vi "Settings Dialog.vi"(8 "error in (no error)":errorcluster, 11 "Settings in":T3={"Acquisition"={"State"=enum."Idle S3DK", "Settings"="", "Online"=FALSE, "S3DK"={"Signals"={"Phasor"=[], "Analog"=[], "Digital"=[]}}, "CSV"={"Index"=0, "Parcel Length"=0, "EOF?"=FALSE, "Config"={"Mode"=enum."Full timestamp", "delimiter (\\t)"="\t", "Path"=path "", "Rectangular?"=FALSE}}}, "Logging"={"Logging State"=enum."Idle", "Settings"="", "Buffer"={"Index"=0, "Size"=15000, "Samples"=0, "Ordered ?"=FALSE}}, "Processing"={"Settings"="", "Parameters"={"Index"=0, "Size"=0, "Samples"=0, "Ordered ?"=FALSE}, "Refresh Rate"=0}}) -> (0 "error out":errorcluster, 1 "Changed?":bool, 2 "UI Refresh Needed?":bool, 3 "Settings out":T3={"Acquisition"={"State"=enum."Idle S3DK", "Settings"="", "Online"=FALSE, "S3DK"={"Signals"={"Phasor"=[], "Analog"=[], "Digital"=[]}}, "CSV"={"Index"=0, "Parcel Length"=0, "EOF?"=FALSE, "Config"={"Mode"=enum."Full timestamp", "delimiter (\\t)"="\t", "Path"=path "", "Rectangular?"=FALSE}}}, "Logging"={"Logging State"=enum."Idle", "Settings"="", "Buffer"={"Index"=0, "Size"=15000, "Samples"=0, "Ordered ?"=FALSE}}, "Processing"={"Settings"="", "Parameters"={"Index"=0, "Size"=0, "Samples"=0, "Ordered ?"=FALSE}, "Refresh Rate"=0}})   [LabVIEW 2017, in "Settings.lvlib"]
doc: "Dialog for selecting user specified settings."
uses:
  Settings.lvlib
  Settings.ctl
  acquisition/Acquisition Settings.ctl
  acquisition/Acquisition State.ctl
  libs/CSV Reader/Mode CSV reader.ctl
  logging/Logging Configuration.ctl
  logging/Logging State.ctl
  libs/PMU Buffer/Buffer Settings.ctl
  processing/Processing Settings.ctl
  acquisition/Acquisition.lvlib
  logging/Logging.lvlib
  processing/Processing.lvlib
  libs/PMU Buffer/PMU data buffer.lvlib
panel:
  in  "Restore Default":bool
  in  "CSV":T2={"Mode"=enum."Full timestamp", "delimiter (\\t)"=";", "Path"=path "", "Rectangular?"=FALSE}
  in  "Online?":bool
  in  "Parcel Length":i32=20
  in  "Refresh Rate":u32(ring)=1000 caption="Hz" items=["1"=1000, "5"=200, "10"=100, "25"=40, "50"=20]
  in  "Buffer Size":i32=3000
  in  "Cancel Button":bool
  in  "OK Button":bool
  # "Non visible portion of dialog (needed for connector pane)."
  # "Buffer Paremeters"
  # "Buffer Paremeters"
  # "Buffer Paremeters"
  # "Buffer Paremeters"
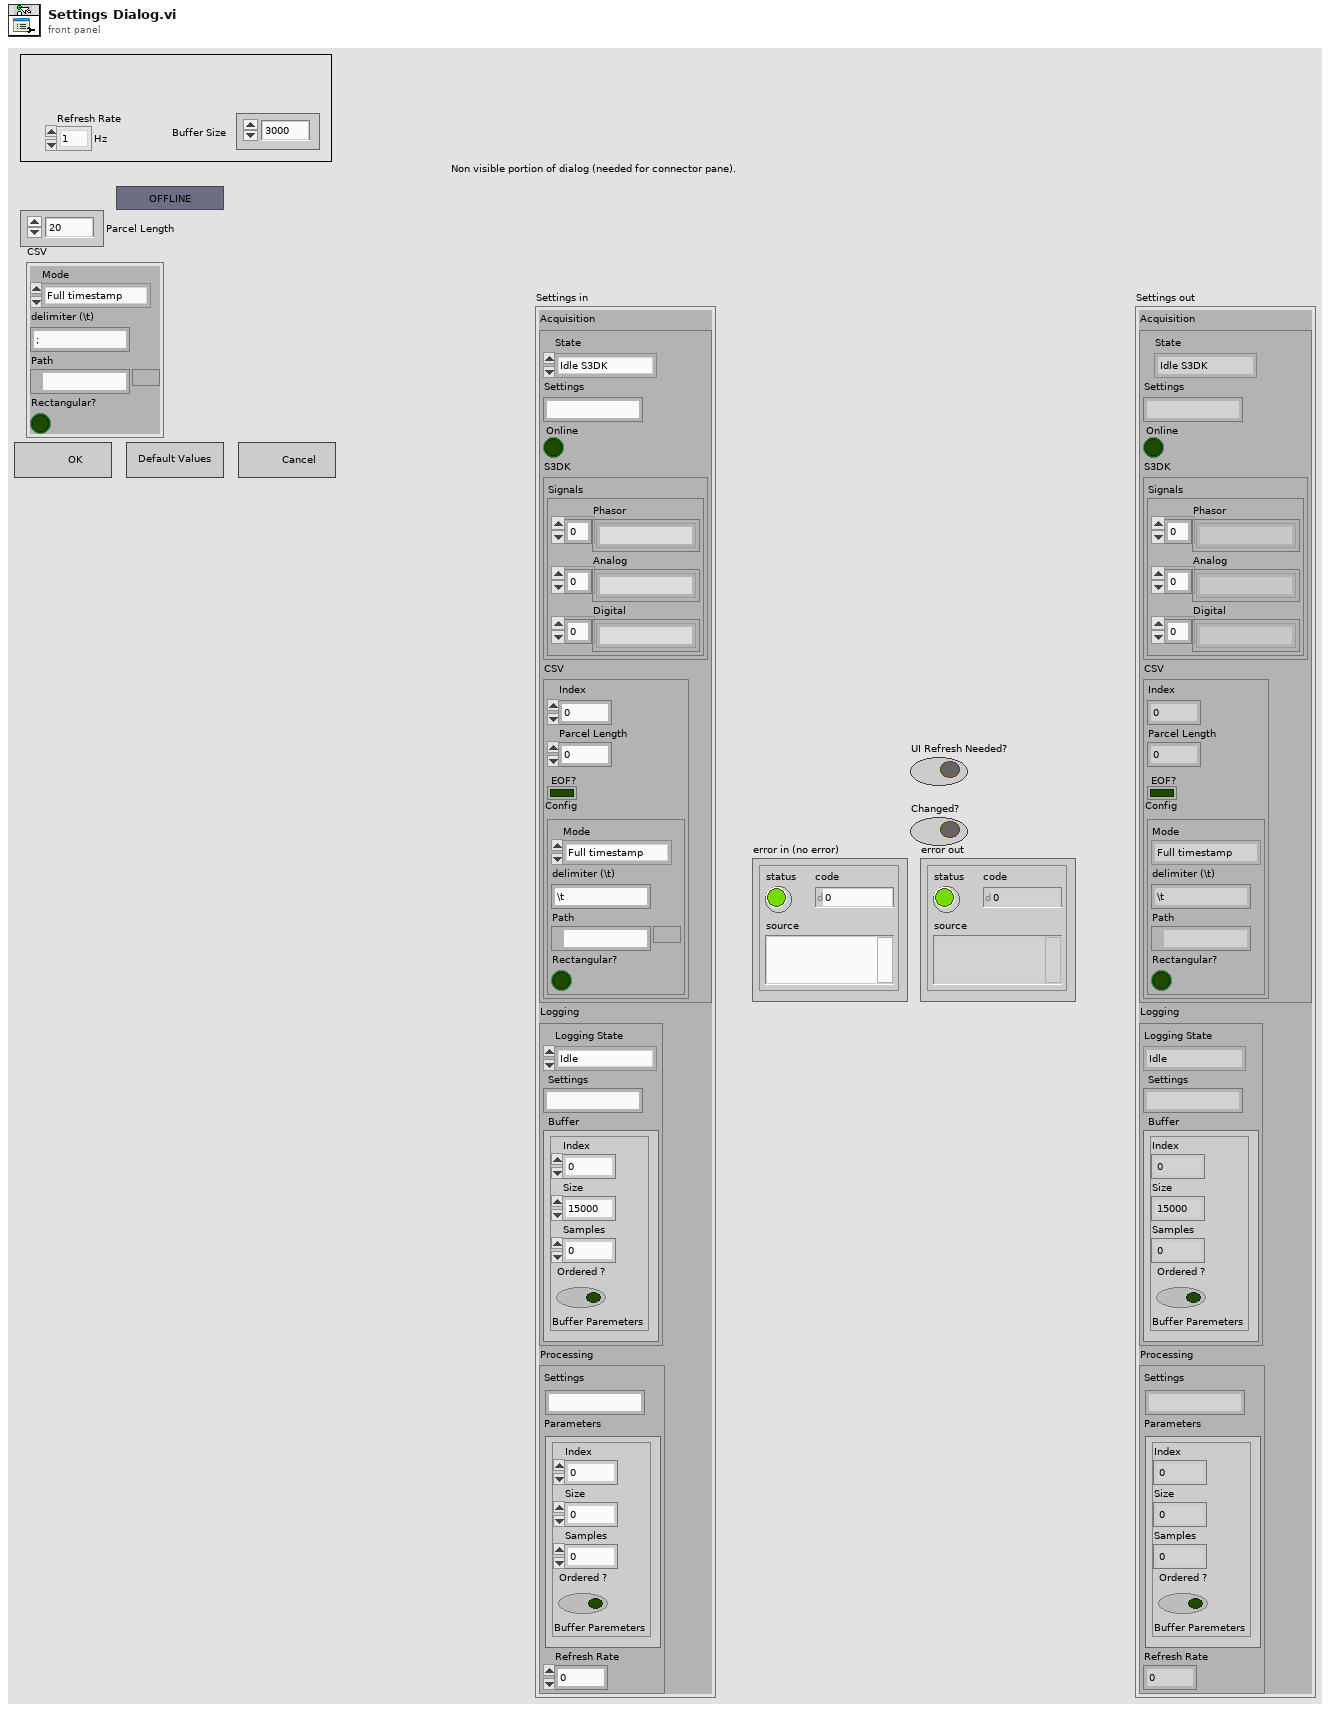
[diagram p1: front panel]
types:
  T1 = typedef "Mode CSV reader.ctl" = enum16{"Full timestamp", "Relative Time", "Seconds Time"}
  T2 = cluster{"Mode":T1, "delimiter (\\t)":string, "Path":path, "Rectangular?":bool}
  T3 = typedef "Settings.lvlib/Settings.ctl" = cluster{"Acquisition":T4, "Logging":T6, "Processing":T9}
  T4 = typedef "Acquisition.lvlib/Acquisition Settings.ctl" = cluster{"State":T5, "Settings":string, "Online":bool, "S3DK":cluster{"Signals":cluster{"Phasor":string[], "Analog":string[], "Digital":string[]}}, "CSV":cluster{"Index":i32, "Parcel Length":i32, "EOF?":bool, "Config":cluster{"Mode":T1, "delimiter (\\t)":string, "Path":path, "Rectangular?":bool}}}
  T5 = typedef "Acquisition.lvlib/Acquisition State.ctl" = enum16{"Idle", "Idle S3DK", "Acquiring S3DK", "Idle CSV", "Acquiring CSV"}
  T6 = typedef "Logging.lvlib/Logging Configuration.ctl" = cluster{"Logging State":T7, "Settings":string, "Buffer":T8}
  T7 = typedef "Logging.lvlib/Logging State.ctl" = enum16{"Idle", "Logging"}
  T8 = typedef "PMU data buffer.lvlib/Buffer Settings.ctl" = cluster{"Index":i32, "Size":i32, "Samples":i32, "Ordered ?":bool}
  T9 = typedef "Processing.lvlib/Processing Settings.ctl" = cluster{"Settings":string, "Parameters":T8, "Refresh Rate":u32}
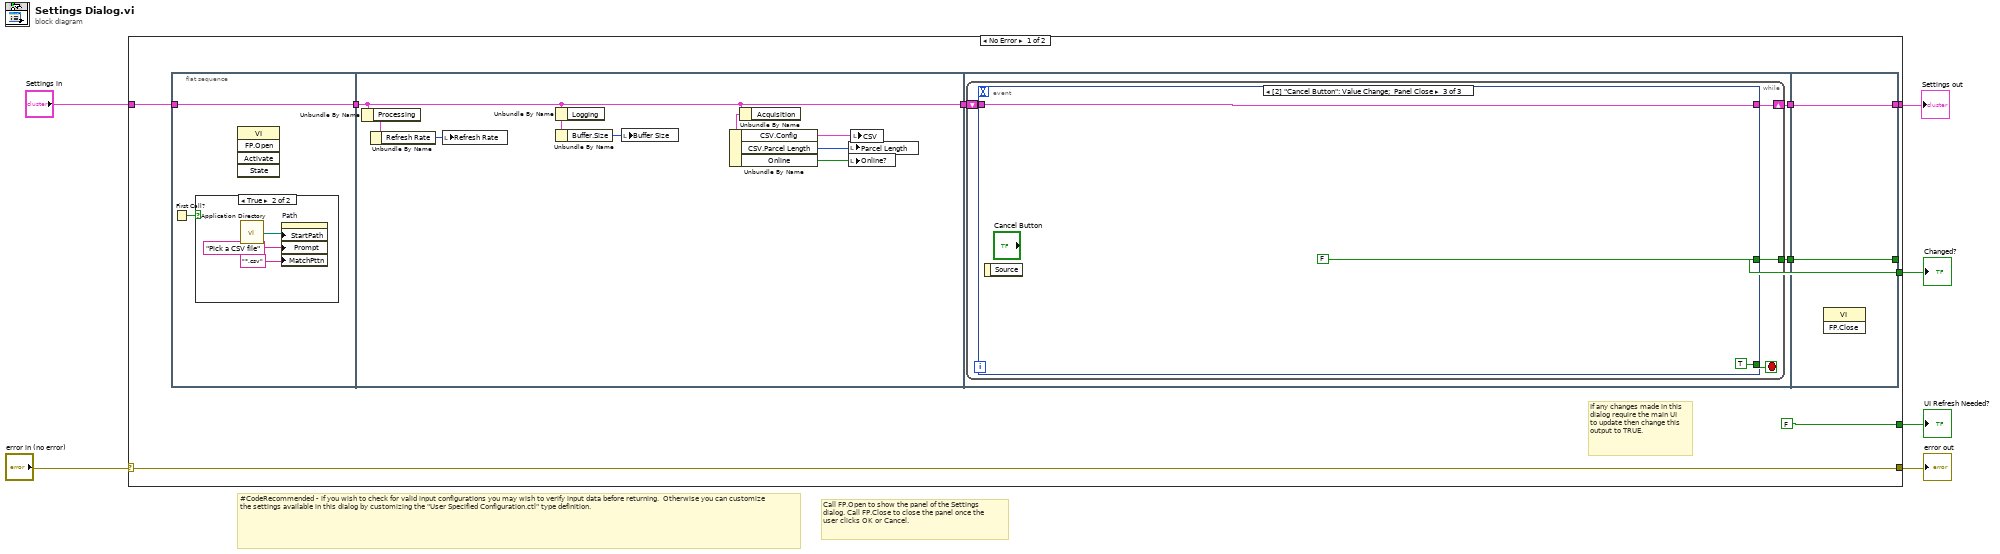
[diagram p0: block diagram]
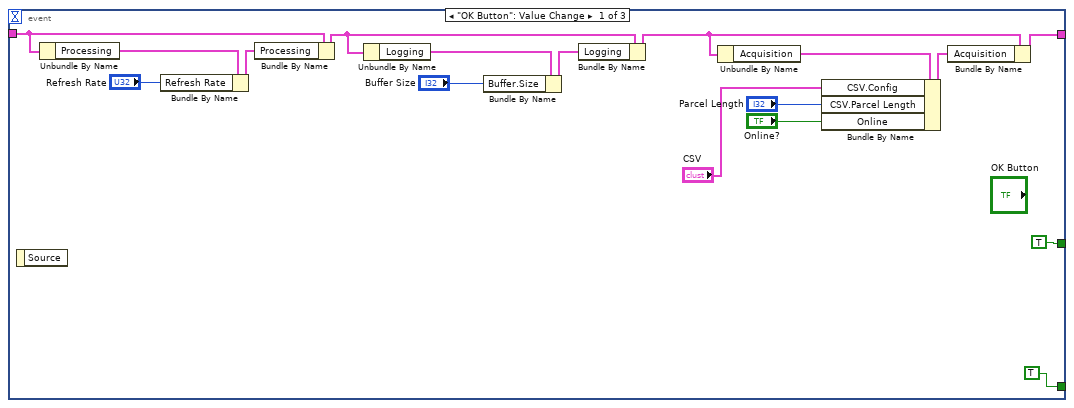
[diagram p3: hidden frame]
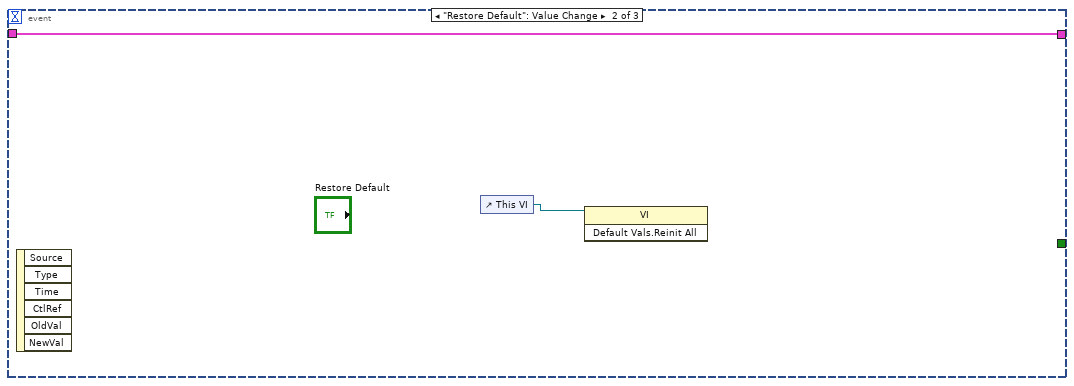
[diagram p4: hidden frame]
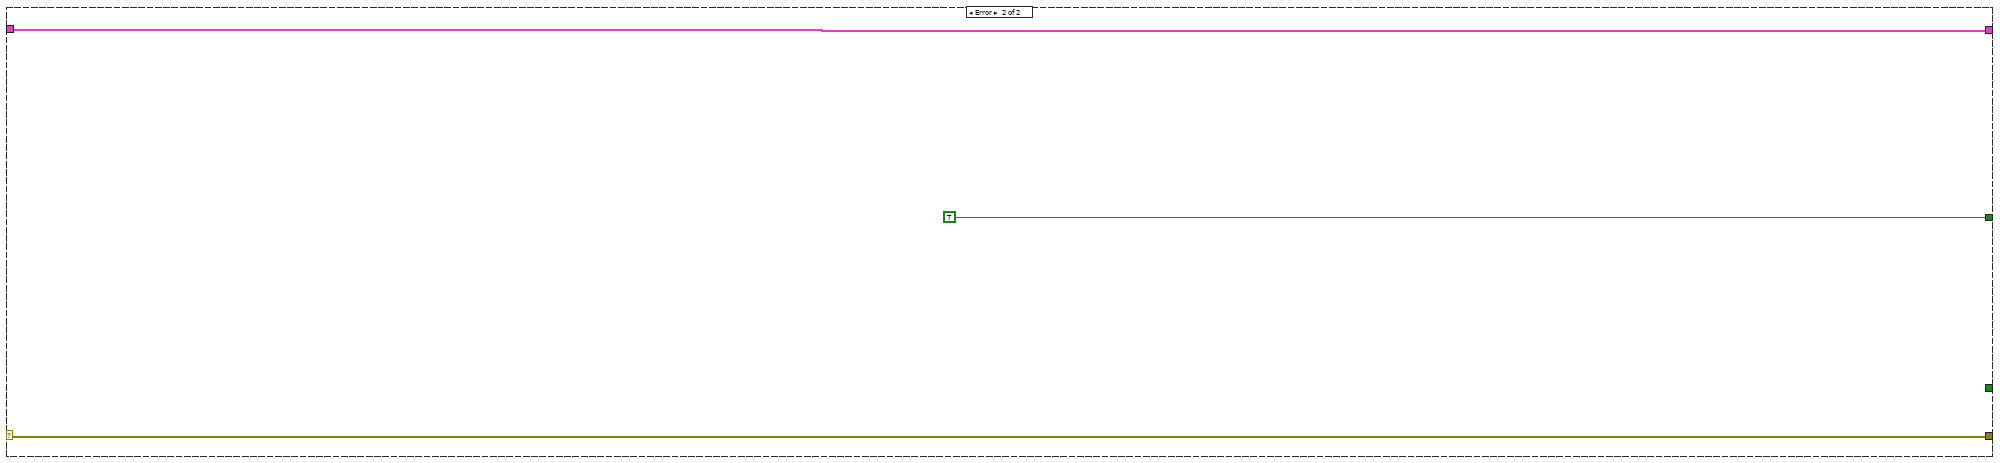
[diagram p5: hidden frame]
diagram:
  # "Call FP.Open to show the panel of the Settings dialog. Call FP.Close to close the panel once the user clicks OK or Cancel."
  # "#CodeRecommended - if you wish to check for valid input configurations you may wish to verify input data before returning.  Otherwise you can customize the settings available in this dialog by customizing the \"User Specified Configuration.ctl\" type definition."
  n1 = case shown="No Error" "error in (no error)" {
    selector: "error in (no error)" -> [w15 w63]
    tunnel: [w15 w63] -> w5
    tunnel: "Settings in" -> [w11 w62]
    tunnel: [w12 w62] -> w3
    tunnel: [FALSE ("UI Refresh Needed?") _] -> w2
    tunnel: [w13 TRUE ("UI Refresh Needed?")] -> w1
    frame No Error {
      # "If any changes made in this dialog require the main UI to update then change this output to TRUE."
      n2 = flat-sequence {
        tunnel: w11 -> [w17]
        tunnel: [w17] -> w8
        tunnel: w8 -> [w24]
        tunnel: [w24] -> w7
        tunnel: w7 -> [w30]
        tunnel: [w32] -> w10
        tunnel: [w31] -> w9
        tunnel: [w59] -> w12
        tunnel: [w60] -> w13
        tunnel: w10 -> [w60]
        tunnel: w9 -> [w59]
        frame #0 {
          n3 = First Call?() -> (First Call?: T/F=w16:bool)
          n4 = case shown="True" w16 {
            frame False {
            }
            frame True {
              n5 = call <vilib>:"Application Directory.vi"() -> ("Application Directory"=w20:path)
              n6 = property on="Path" class="Path"("StartPath"=w20, "Prompt"="Pick a CSV file" ("Browse Options:Prompt"), "MatchPttn"="*.csv" ("Browse Options:Match Pattern")) -> ()  [unwired: 2 in, 2 out]
            }
          }
          n7 = invoke class="VI" method="FP.Open"() -> ()  [unwired: 5 in, 5 out]
        }
        frame #1 {
          n8 = Unbundle By Name(w24) -> ("Processing"=w29:T9)
          n9 = Unbundle By Name(w29) -> ("Refresh Rate"=w26:u32)
          n10 = local write "Refresh Rate"(w26) -> ()
          n11 = Unbundle By Name(w24) -> ("Logging"=w28:T6)
          n12 = Unbundle By Name(w28) -> ("Buffer.Size"=w27:i32)
          n13 = local write "Buffer Size"(w27) -> ()
          n14 = Unbundle By Name(w24) -> ("Acquisition"=w25:T4)
          n15 = Unbundle By Name(w25) -> ("CSV.Config"=w23:T2, "CSV.Parcel Length"=w22:i32, "Online"=w21:bool)
          n16 = local write "Parcel Length"(w22) -> ()
          n17 = local write "Online?"(w21) -> ()
          n18 = local write "CSV"(w23) -> ()
        }
        frame #2 {
          n19 = while {
            tunnel: [w36] -> w32
            shift-right: [w35] -> w31
            shift-left: w30 -> [w34]
            stop <- w33 stop-if-true
            n20 = event shown="[2] \"Cancel Button\": Value Change;  Panel Close" {
              selector: _ -> [_ _ _]
              dyn-events: _ -> [_ _ _]
              timeout: _ -> [_ _ _]
              tunnel: [w40 w55 w58] -> w35
              tunnel: w34 -> [w50 w55 w58]
              tunnel: [TRUE ("UI Refresh Needed?") _ FALSE ("UI Refresh Needed?")] -> w36
              tunnel: [TRUE ("UI Refresh Needed?") _ TRUE ("UI Refresh Needed?")] -> w33
              event "OK Button": Value Change {
                n21 = event-data() -> ()  [unwired: 1 in, 1 out]
                n22 = Unbundle By Name(w50) -> ("Processing"=w52:T9)
                n23 = Bundle By Name(cluster=w52, "Refresh Rate"="Refresh Rate") -> (w51:T9)
                n24 = Bundle By Name(cluster=w50, "Processing"=w51) -> (w44:T3)
                n25 = Unbundle By Name(w44) -> ("Logging"=w47:T6)
                n26 = Bundle By Name(cluster=w47, "Buffer.Size"="Buffer Size") -> (w48:T6)
                n27 = Bundle By Name(cluster=w44, "Logging"=w48) -> (w42:T3)
                n28 = Unbundle By Name(w42) -> ("Acquisition"=w46:T4)
                n29 = Bundle By Name(cluster=w46, "CSV.Config"="CSV", "CSV.Parcel Length"="Parcel Length", "Online"="Online?") -> (w45:T4)
                n30 = Bundle By Name(cluster=w42, "Acquisition"=w45) -> (w40:T3)
              }
              event "Restore Default": Value Change {
                n31 = event-data() -> ()  [unwired: 1 in, 6 out]
                n32 = control-ref of="This VI"() -> (w54:refnum<vi>)
                n33 = invoke class="VI" method="Default Vals.Reinit All"(reference=w54) -> ()  [unwired: 2 in, 3 out]
              }
              event "Cancel Button": Value Change; Panel Close {
                n34 = event-data() -> ()  [unwired: 1 in, 1 out]
              }
            }
          }
        }
        frame #3 {
          n35 = invoke class="VI" method="FP.Close"() -> ()  [unwired: 3 in, 3 out]
        }
      }
    }
    frame Error {
    }
  }
  "UI Refresh Needed?" <- w2
  "error out" <- w5
  "Settings out" <- w3
  "Changed?" <- w1
